vi "Get Parameter.vi"(8 "error in (no error)":errorcluster, 11 "ParameterDevice in":refnum<class "ParameterDevice.lvclass">) -> (0 "error out":errorcluster, 2 "Parameter":refnum<class "AbstractData.lvclass">, 3 "ParameterDevice out":refnum<class "ParameterDevice.lvclass">)   [LabVIEW 2014, in "ParameterDevice.lvclass"]
uses:
  ParameterDevice.lvclass
  Model/Data/AbstractData/AbstractData.lvclass
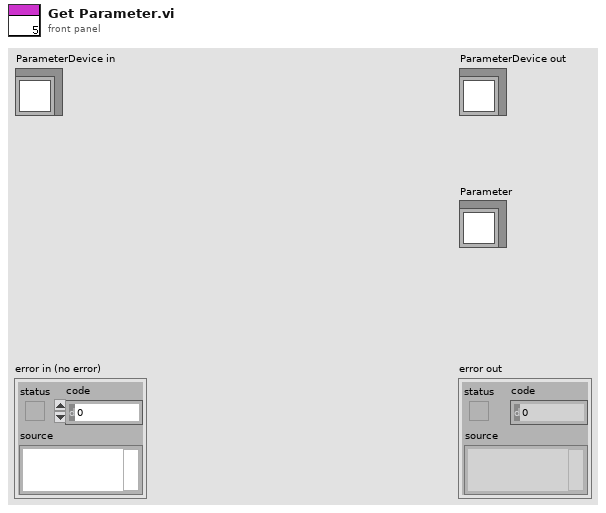
[diagram p1: front panel]
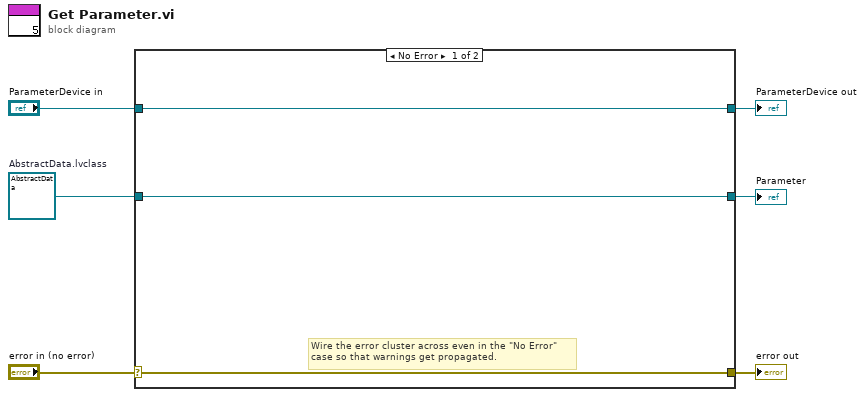
[diagram p0: block diagram]
diagram:
  w1 = refnum<class "AbstractData.lvclass"> refnum  # AbstractData.lvclass
  n1 = case shown="No Error" "error in (no error)" {
    selector: "error in (no error)" -> [w8 w12]
    tunnel: [w8 w12] -> w5
    tunnel: [w9 w11] -> w3
    tunnel: "ParameterDevice in" -> [w9 w11]
    tunnel: [w7 w10] -> w2
    tunnel: w1 -> [w7 w10]
    frame No Error {
      # "Wire the error cluster across even in the \"No Error\"\ncase so that warnings get propagated."
    }
    frame Error {
    }
  }
  "error out" <- w5
  "ParameterDevice out" <- w3
  "Parameter" <- w2
